vi "4-Graph of Trigonometric Functions.vi"() -> ()   [LabVIEW 2020]
panel:
  out "Multiple Signal Display":cluster{"a":dbl, "b":dbl}(graph)
  out "Single Signal Display(Sum)":dbl(graph)
  in  "w2":dbl=30.0
  in  "f2":dbl=20.0
  in  "f1":dbl=40.0
  in  "f":dbl=60.0
  in  "w1":dbl=20.0
  in  "w":dbl=10.0
  in  "B":dbl=2.0
  in  "A":dbl=1.0
  in  "stop":bool
  in  "Trigonomic Function Selector":T1(ring)
  # "Amplitude"
  # "Frequency"
  # "Phase"
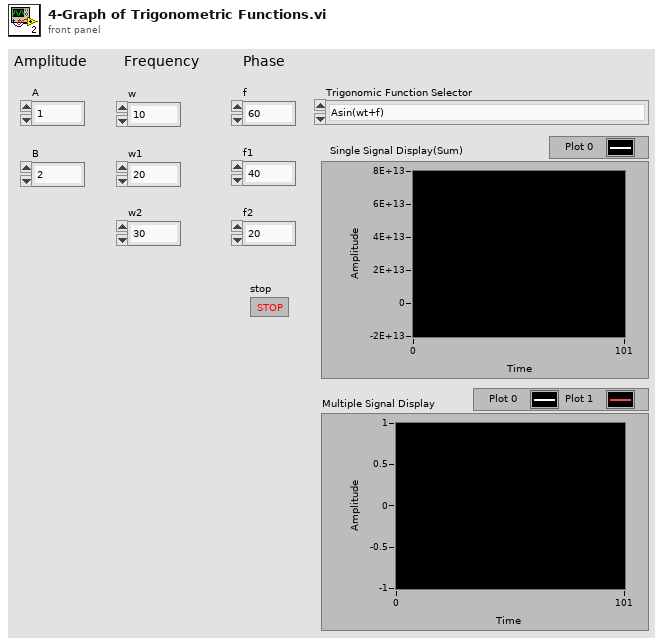
[diagram p1: front panel]
types:
  T1 = enum16{"Asin(wt+f)", "Acos(wt+f)", "Atan(wt+f)", "Acot(wt+f)", "Asin(w1t+f1)+Bcos(w2t+f2)", "Atan(w1t+f1)+Bcot(w2t+f2)"}
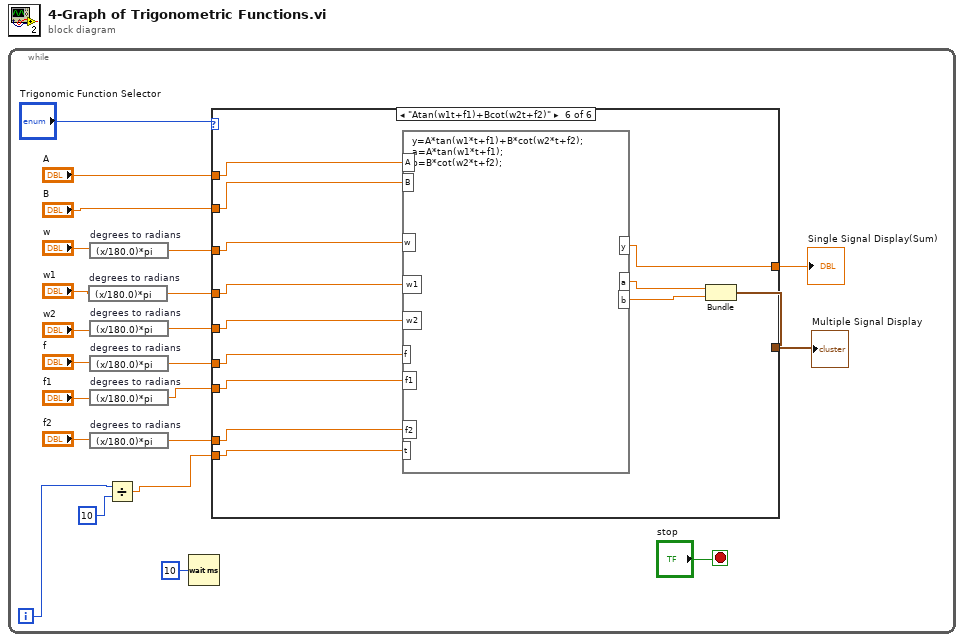
[diagram p0: block diagram]
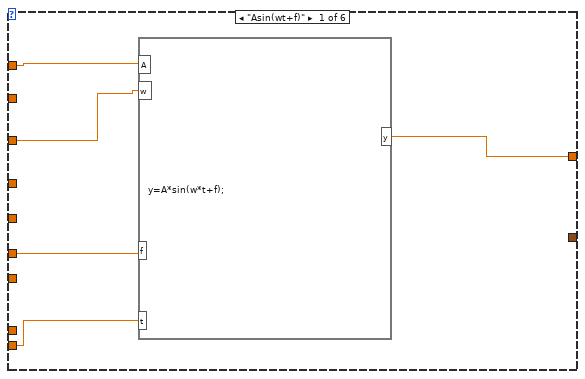
[diagram p2: hidden frame]
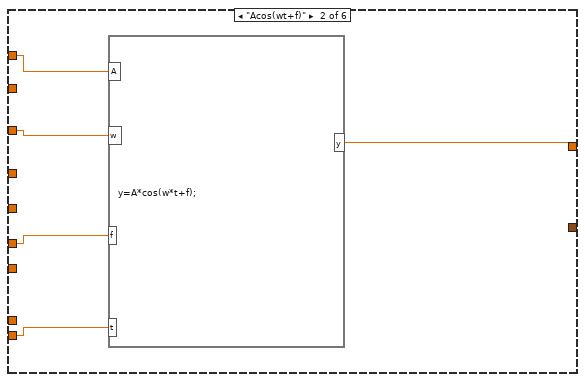
[diagram p3: hidden frame]
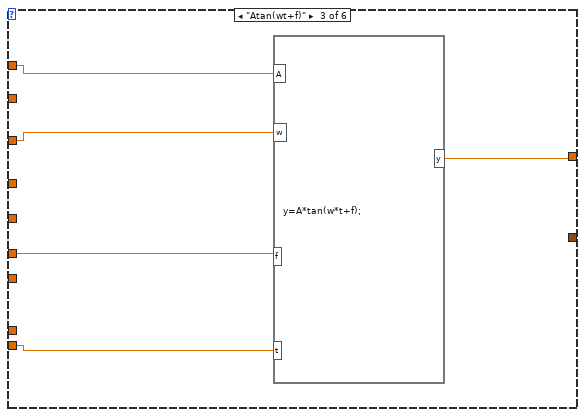
[diagram p4: hidden frame]
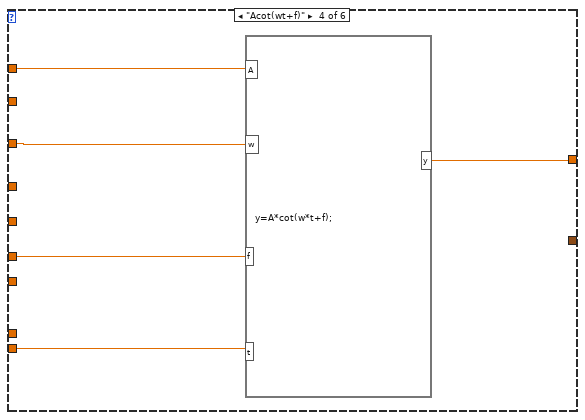
[diagram p5: hidden frame]
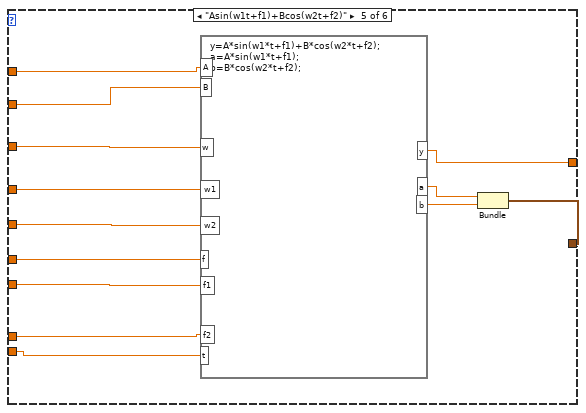
[diagram p6: hidden frame]
diagram:
  n1 = while {
    i -> [w3]
    stop <- "stop" stop-if-true
    n2 = expression code="(x/180.0)*pi" "degrees to radians"("w1") -> (w9:dbl)
    n3 = expression code="(x/180.0)*pi" "degrees to radians"("w") -> (w8:dbl)
    n4 = expression code="(x/180.0)*pi" "degrees to radians"("w2") -> (w10:dbl)
    n5 = expression code="(x/180.0)*pi" "degrees to radians"("f") -> (w11:dbl)
    n6 = expression code="(x/180.0)*pi" "degrees to radians"("f1") -> (w12:dbl)
    n7 = expression code="(x/180.0)*pi" "degrees to radians"("f2") -> (w13:dbl)
    n8 = Divide(x=w3, y=10) -> (x/y=w1:dbl)
    n9 = Wait (ms)(milliseconds to wait=u32 10) -> ()  [unwired: 1 out]
    n10 = case shown="\"Atan(w1t+f1)+Bcot(w2t+f2)\"" "Trigonomic Function Selector" {
      tunnel: w1 -> [w27 w32 w37 w42 w55 w56]
      tunnel: w13 -> [_ _ _ _ w52 w57]
      tunnel: w12 -> [_ _ _ _ w51 w58]
      tunnel: w11 -> [w25 w29 w34 w39 w50 w59]
      tunnel: w10 -> [_ _ _ _ w49 w60]
      tunnel: w9 -> [_ _ _ _ w48 w61]
      tunnel: w8 -> [w23 w30 w35 w40 w47 w62]
      tunnel: "B" -> [_ _ _ _ w46 w63]
      tunnel: "A" -> [w26 w31 w36 w41 w45 w64]
      tunnel: [w24 w28 w33 w38 w44 w65] -> w5
      tunnel: [_ _ _ _ w43 w66] -> w4
      frame "Asin(wt+f)" {
        n11 = formula code="y=A*sin(w*t+f);"("t"=w27, "A"=w26, "w"=w23, "f"=w25) -> ("y"=w24:dbl)
      }
      frame "Acos(wt+f)" {
        n12 = formula code="y=A*cos(w*t+f);"("A"=w31, "f"=w29, "w"=w30, "t"=w32) -> ("y"=w28:dbl)
      }
      frame "Atan(wt+f)" {
        n13 = formula code="y=A*tan(w*t+f);"("A"=w36, "w"=w35, "f"=w34, "t"=w37) -> ("y"=w33:dbl)
      }
      frame "Acot(wt+f)" {
        n14 = formula code="y=A*cot(w*t+f);"("A"=w41, "w"=w40, "f"=w39, "t"=w42) -> ("y"=w38:dbl)
      }
      frame "Asin(w1t+f1)+Bcos(w2t+f2)" {
        n15 = formula code="y=A*sin(w1*t+f1)+B*cos(w2*t+f2);\na=A*sin(w1*t+f1);\nb=B*cos(w2*t+f2);"("t"=w55, "A"=w45, "B"=w46, "w"=w47, "w1"=w48, "w2"=w49, "f"=w50, "f1"=w51, "f2"=w52) -> ("a"=w53:dbl, "b"=w54:dbl, "y"=w44:dbl)
        n16 = Bundle("a"=w53, "b"=w54) -> (w43:cluster{"a":dbl, "b":dbl})  [unwired: 1 in]
      }
      frame "Atan(w1t+f1)+Bcot(w2t+f2)" {
        n17 = formula code="y=A*tan(w1*t+f1)+B*cot(w2*t+f2);\na=A*tan(w1*t+f1);\nb=B*cot(w2*t+f2);"("t"=w56, "A"=w64, "B"=w63, "w"=w62, "w1"=w61, "w2"=w60, "f"=w59, "f1"=w58, "f2"=w57) -> ("a"=w68:dbl, "b"=w67:dbl, "y"=w65:dbl)
        n18 = Bundle("a"=w68, "b"=w67) -> (w66:cluster{"a":dbl, "b":dbl})  [unwired: 1 in]
      }
    }
    "Single Signal Display(Sum)" <- w5
    "Multiple Signal Display" <- w4
  }
